vi "Methods to Tree Arr.vi"(7 "Action":T1, 10 "Class":string, 11 "Methods[]":T3(array[cluster])) -> (3 "Properties for Tree Out":T2(array[cluster]))   [LabVIEW 2023] (continued)
Name (localized)"="SceneObject"}, "Method Info"={"Unique ID string"="2d87741e", "Data name"="Light.Set State", "Short name (localized)"="Light.Set State", "Long name (localized)"="Light:Set State"}, "Method Flags"={"IsDeprecated"=FALSE, "IsPrivate"=FALSE, "IsScripting"=FALSE, "IsNotInRun-Time"=FALSE}, "Divider"=FALSE}, {"Class Info"={"Unique ID string"="105", "Parent ID string"="104", "Class Name (unlocalized)"="SceneObject", "Class Name (localized)"="SceneObject"}, "Method Info"={"Unique ID string"="2d87741f", "Data name"="Clip Plane.Get State", "Short name (localized)"="Clip Plane.Get State", "Long name (localized)"="Clip Plane:Get State"}, "Method Flags"={"IsDeprecated"=FALSE, "IsPrivate"=FALSE, "IsScripting"=FALSE, "IsNotInRun-Time"=FALSE}, "Divider"=FALSE}, {"Class Info"={"Unique ID string"="105", "Parent ID string"="104", "Class Name (unlocalized)"="SceneObject", "Class Name (localized)"="SceneObject"}, "Method Info"={"Unique ID string"="2d877420", "Data name"="Clip Plane.Set State", "Short name (localized)"="Clip Plane.Set State", "Long name (localized)"="Clip Plane:Set State"}, "Method Flags"={"IsDeprecated"=FALSE, "IsPrivate"=FALSE, "IsScripting"=FALSE, "IsNotInRun-Time"=FALSE}, "Divider"=FALSE}, {"Class Info"={"Unique ID string"="105", "Parent ID string"="104", "Class Name (unlocalized)"="SceneObject", "Class Name (localized)"="SceneObject"}, "Method Info"={"Unique ID string"="2d877421", "Data name"="Object.Get Object", "Short name (localized)"="Object.Get Object", "Long name (localized)"="Object:Get Object"}, "Method Flags"={"IsDeprecated"=FALSE, "IsPrivate"=FALSE, "IsScripting"=FALSE, "IsNotInRun-Time"=FALSE}, "Divider"=FALSE}, {"Class Info"={"Unique ID string"="105", "Parent ID string"="104", "Class Name (unlocalized)"="SceneObject", "Class Name (localized)"="SceneObject"}, "Method Info"={"Unique ID string"="2d877423", "Data name"="Texture.Set Texture", "Short name (localized)"="Texture.Set Texture", "Long name (localized)"="Texture:Set Texture"}, "Method Flags"={"IsDeprecated"=FALSE, "IsPrivate"=FALSE, "IsScripting"=FALSE, "IsNotInRun-Time"=FALSE}, "Divider"=FALSE}, {"Class Info"={"Unique ID string"="105", "Parent ID string"="104", "Class Name (unlocalized)"="SceneObject", "Class Name (localized)"="SceneObject"}, "Method Info"={"Unique ID string"="2d877424", "Data name"="Texture.RemoveTexture", "Short name (localized)"="Texture.RemoveTexture", "Long name (localized)"="Texture:Remove Texture"}, "Method Flags"={"IsDeprecated"=FALSE, "IsPrivate"=FALSE, "IsScripting"=FALSE, "IsNotInRun-Time"=FALSE}, "Divider"=FALSE}, {"Class Info"={"Unique ID string"="105", "Parent ID string"="104", "Class Name (unlocalized)"="SceneObject", "Class Name (localized)"="SceneObject"}, "Method Info"={"Unique ID string"="2d877425", "Data name"="Light.Add Light", "Short name (localized)"="Light.Add Light", "Long name (localized)"="Light:Add Light"}, "Method Flags"={"IsDeprecated"=FALSE, "IsPrivate"=FALSE, "IsScripting"=FALSE, "IsNotInRun-Time"=FALSE}, "Divider"=FALSE}, {"Class Info"={"Unique ID string"="105", "Parent ID string"="104", "Class Name (unlocalized)"="SceneObject", "Class Name (localized)"="SceneObject"}, "Method Info"={"Unique ID string"="2d877426", "Data name"="Clip Plane.Add Clip Plane", "Short name (localized)"="Clip Plane.Add Clip Plane", "Long name (localized)"="Clip Plane:Add Clip Plane"}, "Method Flags"={"IsDeprecated"=FALSE, "IsPrivate"=FALSE, "IsScripting"=FALSE, "IsNotInRun-Time"=FALSE}, "Divider"=FALSE}, {"Class Info"={"Unique ID string"="105", "Parent ID string"="104", "Class Name (unlocalized)"="SceneObject", "Class Name (localized)"="SceneObject"}, "Method Info"={"Unique ID string"="2d877427", "Data name"="Transformation.Get Rotation", "Short name (localized)"="Transformation.Get Rotation", "Long name (localized)"="Transformation:Get Rotation"}, "Method Flags"={"IsDeprecated"=FALSE, "IsPrivate"=FALSE, "IsScripting"=FALSE, "IsNotInRun-Time"=FALSE}, "Divider"=FALSE}, {"Class Info"={"Unique ID string"="105", "Parent ID string"="104", "Class Name (unlocalized)"="SceneObject", "Class Name (localized)"="SceneObject"}, "Method Info"={"Unique ID string"="2d877428", "Data name"="Transformation.Get Translation", "Short name (localized)"="Transformation.Get Translation", "Long name (localized)"="Transformation:Get Translation"}, "Method Flags"={"IsDeprecated"=FALSE, "IsPrivate"=FALSE, "IsScripting"=FALSE, "IsNotInRun-Time"=FALSE}, "Divider"=FALSE}, {"Class Info"={"Unique ID string"="105", "Parent ID string"="104", "Class Name (unlocalized)"="SceneObject", "Class Name (localized)"="SceneObject"}, "Method Info"={"Unique ID string"="2d877429", "Data name"="Transformation.Get Scale", "Short name (localized)"="Transformation.Get Scale", "Long name (localized)"="Transformation:Get Scale"}, "Method Flags"={"IsDeprecated"=FALSE, "IsPrivate"=FALSE, "IsScripting"=FALSE, "IsNotInRun-Time"=FALSE}, "Divider"=FALSE}, {"Class Info"={"Unique ID string"="105", "Parent ID string"="104", "Class Name (unlocalized)"="SceneObject", "Class Name (localized)"="SceneObject"}, "Method Info"={"Unique ID string"="2d87742a", "Data name"="Light.Get Light", "Short name (localized)"="Light.Get Light", "Long name (localized)"="Light:Get Light"}, "Method Flags"={"IsDeprecated"=FALSE, "IsPrivate"=FALSE, "IsScripting"=FALSE, "IsNotInRun-Time"=FALSE}, "Divider"=FALSE}, {"Class Info"={"Unique ID string"="105", "Parent ID string"="104", "Class Name (unlocalized)"="SceneObject", "Class Name (localized)"="SceneObject"}, "Method Info"={"Unique ID string"="2d87742b", "Data name"="Clip Plane.Get Clip", "Short name (localized)"="Clip Plane.Get Clip", "Long name (localized)"="Clip Plane:Get Clip Plane"}, "Method Flags"={"IsDeprecated"=FALSE, "IsPrivate"=FALSE, "IsScripting"=FALSE, "IsNotInRun-Time"=FALSE}, "Divider"=FALSE}, {"Class Info"={"Unique ID string"="105", "Parent ID string"="104", "Class Name (unlocalized)"="SceneObject", "Class Name (localized)"="SceneObject"}, "Method Info"={"Unique ID string"="2d87742c", "Data name"="Light.Remove Light", "Short name (localized)"="Light.Remove Light", "Long name (localized)"="Light:Remove Light"}, "Method Flags"={"IsDeprecated"=FALSE, "IsPrivate"=FALSE, "IsScripting"=FALSE, "IsNotInRun-Time"=FALSE}, "Divider"=FALSE}, {"Class Info"={"Unique ID string"="105", "Parent ID string"="104", "Class Name (unlocalized)"="SceneObject", "Class Name (localized)"="SceneObject"}, "Method Info"={"Unique ID string"="2d87742d", "Data name"="Clip Plane.Remove Clip", "Short name (localized)"="Clip Plane.Remove Clip", "Long name (localized)"="Clip Plane:Remove Clip Plane"}, "Method Flags"={"IsDeprecated"=FALSE, "IsPrivate"=FALSE, "IsScripting"=FALSE, "IsNotInRun-Time"=FALSE}, "Divider"=FALSE}, {"Class Info"={"Unique ID string"="105", "Parent ID string"="104", "Class Name (unlocalized)"="SceneObject", "Class Name (localized)"="SceneObject"}, "Method Info"={"Unique ID string"="2d87742e", "Data name"="Light.Light Count", "Short name (localized)"="Light.Light Count", "Long name (localized)"="Light:Light Count"}, "Method Flags"={"IsDeprecated"=FALSE, "IsPrivate"=FALSE, "IsScripting"=FALSE, "IsNotInRun-Time"=FALSE}, "Divider"=FALSE}, {"Class Info"={"Unique ID string"="105", "Parent ID string"="104", "Class Name (unlocalized)"="SceneObject", "Class Name (localized)"="SceneObject"}, "Method Info"={"Unique ID string"="2d87742f", "Data name"="Clip Plane.Clip Count", "Short name (localized)"="Clip Plane.Clip Count", "Long name (localized)"="Clip Plane:Clip Plane Count"}, "Method Flags"={"IsDeprecated"=FALSE, "IsPrivate"=FALSE, "IsScripting"=FALSE, "IsNotInRun-Time"=FALSE}, "Divider"=FALSE}, {"Class Info"={"Unique ID string"="105", "Parent ID string"="104", "Class Name (unlocalized)"="SceneObject", "Class Name (localized)"="SceneObject"}, "Method Info"={"Unique ID string"="2d877430", "Data name"="Object.FindObject", "Short name (localized)"="Object.FindObject", "Long name (localized)"="Object:Find Object"}, "Method Flags"={"IsDeprecated"=FALSE, "IsPrivate"=FALSE, "IsScripting"=FALSE, "IsNotInRun-Time"=FALSE}, "Divider"=FALSE}, {"Class Info"={"Unique ID string"="105", "Parent ID string"="104", "Class Name (unlocalized)"="SceneObject", "Class Name (localized)"="SceneObject"}, "Method Info"={"Unique ID string"="2d877431", "Data name"="Set Drawable", "Short name (localized)"="Set Drawable", "Long name (localized)"="Set Drawable"}, "Method Flags"={"IsDeprecated"=FALSE, "IsPrivate"=FALSE, "IsScripting"=FALSE, "IsNotInRun-Time"=FALSE}, "Divider"=FALSE}, {"Class Info"={"Unique ID string"="105", "Parent ID string"="104", "Class Name (unlocalized)"="SceneObject", "Class Name (localized)"="SceneObject"}, "Method Info"={"Unique ID string"="2d877432", "Data name"="SetBillboardParams", "Short name (localized)"="SetBillboardParams", "Long name (localized)"="Set Billboard Params"}, "Method Flags"={"IsDeprecated"=FALSE, "IsPrivate"=FALSE, "IsScripting"=FALSE, "IsNotInRun-Time"=FALSE}, "Divider"=FALSE}, {"Class Info"={"Unique ID string"="105", "Parent ID string"="104", "Class Name (unlocalized)"="SceneObject", "Class Name (localized)"="SceneObject"}, "Method Info"={"Unique ID string"="2d877433", "Data name"="Meshify", "Short name (localized)"="Meshify", "Long name (localized)"="Meshify"}, "Method Flags"={"IsDeprecated"=FALSE, "IsPrivate"=TRUE, "IsScripting"=FALSE, "IsNotInRun-Time"=FALSE}, "Divider"=FALSE}, {"Class Info"={"Unique ID string"="105", "Parent ID string"="104", "Class Name (unlocalized)"="SceneObject", "Class Name (localized)"="SceneObject"}, "Method Info"={"Unique ID string"="2d877434", "Data name"="Bounding.Get Box", "Short name (localized)"="Bounding.Get Box", "Long name (localized)"="Bounding:Get Box"}, "Method Flags"={"IsDeprecated"=FALSE, "IsPrivate"=TRUE, "IsScripting"=FALSE, "IsNotInRun-Time"=FALSE}, "Divider"=FALSE}, {"Class Info"={"Unique ID string"="105", "Parent ID string"="104", "Class Name (unlocalized)"="SceneObject", "Class Name (localized)"="SceneObject"}, "Method Info"={"Unique ID string"="2d877435", "Data name"="Bounding.Get Sphere", "Short name (localized)"="Bounding.Get Sphere", "Long name (localized)"="Bounding:Get Sphere"}, "Method Flags"={"IsDeprecated"=FALSE, "IsPrivate"=TRUE, "IsScripting"=FALSE, "IsNotInRun-Time"=FALSE}, "Divider"=FALSE}, {"Class Info"={"Unique ID string"="111", "Parent ID string"="123", "Class Name (unlocalized)"="SceneTexture", "Class Name (localized)"="SceneTexture"}, "Method Info"={"Unique ID string"="22c3400", "Data name"="Transformation.Rotate", "Short name (localized)"="Transformation.Rotate", "Long name (localized)"="Transformation:Rotate"}, "Method Flags"={"IsDeprecated"=FALSE, "IsPrivate"=FALSE, "IsScripting"=FALSE, "IsNotInRun-Time"=FALSE}, "Divider"=FALSE}, {"Class Info"={"Unique ID string"="111", "Parent ID string"="123", "Class Name (unlocalized)"="SceneTexture", "Class Name (localized)"="SceneTexture"}, "Method Info"={"Unique ID string"="22c3401", "Data name"="Transformation:Translate", "Short name (localized)"="Transformation:Translate", "Long name (localized)"="Transformation:Translate"}, "Method Flags"={"IsDeprecated"=FALSE, "IsPrivate"=FALSE, "IsScripting"=FALSE, "IsNotInRun-Time"=FALSE}, "Divider"=FALSE}, {"Class Info"={"Unique ID string"="111", "Parent ID string"="123", "Class Name (unlocalized)"="SceneTexture", "Class Name (localized)"="SceneTexture"}, "Method Info"={"Unique ID string"="22c3402", "Data name"="Transformation.Scale", "Short name (localized)"="Transformation.Scale", "Long name (localized)"="Transformation:Scale"}, "Method Flags"={"IsDeprecated"=FALSE, "IsPrivate"=FALSE, "IsScripting"=FALSE, "IsNotInRun-Time"=FALSE}, "Divider"=FALSE}, {"Class Info"={"Unique ID string"="111", "Parent ID string"="123", "Class Name (unlocalized)"="SceneTexture", "Class Name (localized)"="SceneTexture"}, "Method Info"={"Unique ID string"="22c3406", "Data name"="Transformation.Clear Transformation", "Short name (localized)"="Transformation.Clear Transformation", "Long name (localized)"="Transformation:Clear Transformation"}, "Method Flags"={"IsDeprecated"=FALSE, "IsPrivate"=FALSE, "IsScripting"=FALSE, "IsNotInRun-Time"=FALSE}, "Divider"=FALSE}, {"Class Info"={"Unique ID string"="111", "Parent ID string"="123", "Class Name (unlocalized)"="SceneTexture", "Class Name (localized)"="SceneTexture"}, "Method Info"={"Unique ID string"="22c3407", "Data name"="Transformation.Set Rotation", "Short name (localized)"="Transformation.Set Rotation", "Long name (localized)"="Transformation:Set Rotation"}, "Method Flags"={"IsDeprecated"=FALSE, "IsPrivate"=FALSE, "IsScripting"=FALSE, "IsNotInRun-Time"=FALSE}, "Divider"=FALSE}, {"Class Info"={"Unique ID string"="111", "Parent ID string"="123", "Class Name (unlocalized)"="SceneTexture", "Class Name (localized)"="SceneTexture"}, "Method Info"={"Unique ID string"="22c3408", "Data name"="Transformation.SetTranslation", "Short name (localized)"="Transformation.SetTranslation", "Long name (localized)"="Transformation:Set Translation"}, "Method Flags"={"IsDeprecated"=FALSE, "IsPrivate"=FALSE, "IsScripting"=FALSE, "IsNotInRun-Time"=FALSE}, "Divider"=FALSE}, {"Class Info"={"Unique ID string"="111", "Parent ID string"="123", "Class Name (unlocalized)"="SceneTexture", "Class Name (localized)"="SceneTexture"}, "Method Info"={"Unique ID string"="22c3409", "Data name"="Transformation.Set Scale", "Short name (localized)"="Transformation.Set Scale", "Long name (localized)"="Transformation:Set Scale"}, "Method Flags"={"IsDeprecated"=FALSE, "IsPrivate"=FALSE, "IsScripting"=FALSE, "IsNotInRun-Time"=FALSE}, "Divider"=FALSE}, {"Class Info"={"Unique ID string"="111", "Parent ID string"="123", "Class Name (unlocalized)"="SceneTexture", "Class Name (localized)"="SceneTexture"}, "Method Info"={"Unique ID string"="22c340a", "Data name"="Transformation.Get Rotation", "Short name (localized)"="Transformation.Get Rotation", "Long name (localized)"="Transformation:Get Rotation"}, "Method Flags"={"IsDeprecated"=FALSE, "IsPrivate"=FALSE, "IsScripting"=FALSE, "IsNotInRun-Time"=FALSE}, "Divider"=FALSE}, {"Class Info"={"Unique ID string"="111", "Parent ID string"="123", "Class Name (unlocalized)"="SceneTexture", "Class Name (localized)"="SceneTexture"}, "Method Info"={"Unique ID string"="22c340b", "Data name"="Transformation.GetTranslation", "Short name (localized)"="Transformation.GetTranslation", "Long name (localized)"="Transformation:Get Translation"}, "Method Flags"={"IsDeprecated"=FALSE, "IsPrivate"=FALSE, "IsScripting"=FALSE, "IsNotInRun-Time"=FALSE}, "Divider"=FALSE}, {"Class Info"={"Unique ID string"="111", "Parent ID string"="123", "Class Name (unlocalized)"="SceneTexture", "Class Name (localized)"="SceneTexture"}, "Method Info"={"Unique ID string"="22c340c", "Data name"="Transformation.Get Scale", "Short name (localized)"="Transformation.Get Scale", "Long name (localized)"="Transformation:Get Scale"}, "Method Flags"={"IsDeprecated"=FALSE, "IsPrivate"=FALSE, "IsScripting"=FALSE, "IsNotInRun-Time"=FALSE}, "Divider"=FALSE}, {"Class Info"={"Unique ID string"="118", "Parent ID string"="112", "Class Name (unlocalized)"="SceneMesh", "Class Name (localized)"="SceneMesh"}, "Method Info"={"Unique ID string"="62a42c00", "Data name"="SetMeshParms", "Short name (localized)"="SetMeshParms", "Long name (localized)"="Set Mesh Parameters"}, "Method Flags"={"IsDeprecated"=FALSE, "IsPrivate"=FALSE, "IsScripting"=FALSE, "IsNotInRun-Time"=FALSE}, "Divider"=FALSE}, {"Class Info"={"Unique ID string"="118", "Parent ID string"="112", "Class Name (unlocalized)"="SceneMesh", "Class Name (localized)"="SceneMesh"}, "Method Info"={"Unique ID string"="62a42c01", "Data name"="ShareArrays", "Short name (localized)"="ShareArrays", "Long name (localized)"="Share Arrays"}, "Method Flags"={"IsDeprecated"=FALSE, "IsPrivate"=FALSE, "IsScripting"=FALSE, "IsNotInRun-Time"=FALSE}, "Divider"=FALSE}, {"Class Info"={"Unique ID string"="118", "Parent ID string"="112", "Class Name (unlocalized)"="SceneMesh", "Class Name (localized)"="SceneMesh"}, "Method Info"={"Unique ID string"="62a42c02", "Data name"="DelaunayMesh", "Short name (localized)"="DelaunayMesh", "Long name (localized)"="Delaunay Mesh"}, "Method Flags"={"IsDeprecated"=FALSE, "IsPrivate"=FALSE, "IsScripting"=FALSE, "IsNotInRun-Time"=FALSE}, "Divider"=FALSE}, {"Class Info"={"Unique ID string"="120", "Parent ID string"="74", "Class Name (unlocalized)"="PropertyFolder", "Class Name (localized)"="PropertyFolder"}, "Method Info"={"Unique ID string"="630d7c00", "Data name"="Add Prop VI", "Short name (localized)"="Add Prop VI", "Long name (localized)"="Add Property VI"}, "Method Flags"={"IsDeprecated"=FALSE, "IsPrivate"=FALSE, "IsScripting"=FALSE, "IsNotInRun-Time"=TRUE}, "Divider"=FALSE}, {"Class Info"={"Unique ID string"="126", "Parent ID string"="80", "Class Name (unlocalized)"="StatechartLibrary", "Class Name (localized)"="StatechartLibrary"}, "Method Info"={"Unique ID string"="18a16402", "Data name"="Generate Code", "Short name (localized)"="Generate Code", "Long name (localized)"="Generate Code"}, "Method Flags"={"IsDeprecated"=FALSE, "IsPrivate"=FALSE, "IsScripting"=FALSE, "IsNotInRun-Time"=TRUE}, "Divider"=FALSE}, {"Class Info"={"Unique ID string"="126", "Parent ID string"="80", "Class Name (unlocalized)"="StatechartLibrary", "Class Name (localized)"="StatechartLibrary"}, "Method Info"={"Unique ID string"="18a16403", "Data name"="Generate Documentation", "Short name (localized)"="Generate Documentation", "Long name (localized)"="Generate Documentation"}, "Method Flags"={"IsDeprecated"=FALSE, "IsPrivate"=FALSE, "IsScripting"=FALSE, "IsNotInRun-Time"=TRUE}, "Divider"=FALSE}, {"Class Info"={"Unique ID string"="129", "Parent ID string"="128", "Class Name (unlocalized)"="SceneText", "Class Name (localized)"="SceneText"}, "Method Info"={"Unique ID string"="c06c00", "Data name"="SetFontName", "Short name (localized)"="SetFontName", "Long name (localized)"="Set Font by Name"}, "Method Flags"={"IsDeprecated"=FALSE, "IsPrivate"=TRUE, "IsScripting"=FALSE, "IsNotInRun-Time"=FALSE}, "Divider"=FALSE}, {"Class Info"={"Unique ID string"="136", "Parent ID string"="6", "Class Name (unlocalized)"="Set", "Class Name (localized)"="Set"}, "Method Info"={"Unique ID string"="4e878c00", "Data name"="ScrollToElement", "Short name (localized)"="ScrollToElement", "Long name (localized)"="Scroll to Element"}, "Method Flags"={"IsDeprecated"=FALSE, "IsPrivate"=FALSE, "IsScripting"=FALSE, "IsNotInRun-Time"=FALSE}, "Divider"=FALSE}, {"Class Info"={"Unique ID string"="137", "Parent ID string"="6", "Class Name (unlocalized)"="Map", "Class Name (localized)"="Map"}, "Method Info"={"Unique ID string"="16099400", "Data name"="ScrollToKey", "Short name (localized)"="ScrollToKey", "Long name (localized)"="Scroll To Key"}, "Method Flags"={"IsDeprecated"=FALSE, "IsPrivate"=FALSE, "IsScripting"=FALSE, "IsNotInRun-Time"=FALSE}, "Divider"=FALSE}, {"Class Info"={"Unique ID string"="16384", "Parent ID string"="16503", "Class Name (unlocalized)"="Diagram", "Class Name (localized)"="Diagram"}, "Method Info"={"Unique ID string"="6d17c800", "Data name"="ObjectFromPoint", "Short name (localized)"="ObjectFromPoint", "Long name (localized)"="Object From Point"}, "Method Flags"={"IsDeprecated"=FALSE, "IsPrivate"=TRUE, "IsScripting"=TRUE, "IsNotInRun-Time"=FALSE}, "Divider"=FALSE}, {"Class Info"={"Unique ID string"="16384", "Parent ID string"="16503", "Class Name (unlocalized)"="Diagram", "Class Name (localized)"="Diagram"}, "Method Info"={"Unique ID string"="6d17c801", "Data name"="CleanUp", "Short name (localized)"="CleanUp", "Long name (localized)"="Clean Up Diagram"}, "Method Flags"={"IsDeprecated"=FALSE, "IsPrivate"=FALSE, "IsScripting"=TRUE, "IsNotInRun-Time"=FALSE}, "Divider"=FALSE}, {"Class Info"={"Unique ID string"="16384", "Parent ID string"="16503", "Class Name (unlocalized)"="Diagram", "Class Name (localized)"="Diagram"}, "Method Info"={"Unique ID string"="6d17c802", "Data name"="CleanUpOptions", "Short name (localized)"="CleanUpOptions", "Long name (localized)"="Default Diagram Clean Up Options"}, "Method Flags"={"IsDeprecated"=FALSE, "IsPrivate"=FALSE, "IsScripting"=TRUE, "IsNotInRun-Time"=FALSE}, "Divider"=FALSE}, {"Class Info"={"Unique ID string"="16384", "Parent ID string"="16503", "Class Name (unlocalized)"="Diagram", "Class Name (localized)"="Diagram"}, "Method Info"={"Unique ID string"="6d17c804", "Data name"="Create from Data Type", "Short name (localized)"="Create from Data Type", "Long name (localized)"="Create from Data Type"}, "Method Flags"={"IsDeprecated"=FALSE, "IsPrivate"=FALSE, "IsScripting"=TRUE, "IsNotInRun-Time"=TRUE}, "Divider"=FALSE}, {"Class Info"={"Unique ID string"="16385", "Parent ID string"="36", "Class Name (unlocalized)"="Terminal", "Class Name (localized)"="Terminal"}, "Method Info"={"Unique ID string"="6349c00", "Data name"="Create Constant", "Short name (localized)"="Create Constant", "Long name (localized)"="Create Constant"}, "Method Flags"={"IsDeprecated"=FALSE, "IsPrivate"=FALSE, "IsScripting"=TRUE, "IsNotInRun-Time"=TRUE}, "Divider"=FALSE}, {"Class Info"={"Unique ID string"="16385", "Parent ID string"="36", "Class Name (unlocalized)"="Terminal", "Class Name (localized)"="Terminal"}, "Method Info"={"Unique ID string"="6349c01", "Data name"="Create Control", "Short name (localized)"="Create Control", "Long name (localized)"="Create Control"}, "Method Flags"={"IsDeprecated"=FALSE, "IsPrivate"=FALSE, "IsScripting"=TRUE, "IsNotInRun-Time"=TRUE}, "Divider"=FALSE}, {"Class Info"={"Unique ID string"="16385", "Parent ID string"="36", "Class Name (unlocalized)"="Terminal", "Class Name (localized)"="Terminal"}, "Method Info"={"Unique ID string"="6349c02", "Data name"="Create Indicator", "Short name (localized)"="Create Indicator", "Long name (localized)"="Create Indicator"}, "Method Flags"={"IsDeprecated"=FALSE, "IsPrivate"=FALSE, "IsScripting"=TRUE, "IsNotInRun-Time"=TRUE}, "Divider"=FALSE}, {"Class Info"={"Unique ID string"="16385", "Parent ID string"="36", "Class Name (unlocalized)"="Terminal", "Class Name (localized)"="Terminal"}, "Method Info"={"Unique ID string"="6349c03", "Data name"="Connect Wire", "Short name (localized)"="Connect Wire", "Long name (localized)"="Connect Wire"}, "Method Flags"={"IsDeprecated"=FALSE, "IsPrivate"=FALSE, "IsScripting"=TRUE, "IsNotInRun-Time"=TRUE}, "Divider"=FALSE}, {"Class Info"={"Unique ID string"="16385", "Parent ID string"="36", "Class Name (unlocalized)"="Terminal", "Class Name (localized)"="Terminal"}, "Method Info"={"Unique ID string"="6349c04", "Data name"="Create Described Wire", "Short name (localized)"="Create Described Wire", "Long name (localized)"="Create Described Wire"}, "Method Flags"={"IsDeprecated"=FALSE, "IsPrivate"=FALSE, "IsScripting"=TRUE, "IsNotInRun-Time"=TRUE}, "Divider"=FALSE}, {"Class Info"={"Unique ID string"="16385", "Parent ID string"="36", "Class Name (unlocalized)"="Terminal", "Class Name (localized)"="Terminal"}, "Method Info"={"Unique ID string"="6349c05", "Data name"="Create Shared Variable Node", "Short name (localized)"="Create Shared Variable Node", "Long name (localized)"="Create Shared Variable Node"}, "Method Flags"={"IsDeprecated"=FALSE, "IsPrivate"=FALSE, "IsScripting"=TRUE, "IsNotInRun-Time"=TRUE}, "Divider"=FALSE}, {"Class Info"={"Unique ID string"="16386", "Parent ID string"="36", "Class Name (unlocalized)"="Constant", "Class Name (localized)"="Constant"}, "Method Info"={"Unique ID string"="634a800", "Data name"="Discon Typedef", "Short name (localized)"="Discon Typedef", "Long name (localized)"="Disconnect From Typedef"}, "Method Flags"={"IsDeprecated"=FALSE, "IsPrivate"=FALSE, "IsScripting"=TRUE, "IsNotInRun-Time"=TRUE}, "Divider"=FALSE}, {"Class Info"={"Unique ID string"="16386", "Parent ID string"="36", "Class Name (unlocalized)"="Constant", "Class Name (localized)"="Constant"}, "Method Info"={"Unique ID string"="634a801", "Data name"="Update Typedef", "Short name (localized)"="Update Typedef", "Long name (localized)"="Update From Typedef"}, "Method Flags"={"IsDeprecated"=FALSE, "IsPrivate"=FALSE, "IsScripting"=TRUE, "IsNotInRun-Time"=TRUE}, "Divider"=FALSE}, {"Class Info"={"Unique ID string"="16386", "Parent ID string"="36", "Class Name (unlocalized)"="Constant", "Class Name (localized)"="Constant"}, "Method Info"={"Unique ID string"="634a802", "Data name"="Change to Control", "Short name (localized)"="Change to Control", "Long name (localized)"="Change to Control"}, "Method Flags"={"IsDeprecated"=FALSE, "IsPrivate"=FALSE, "IsScripting"=TRUE, "IsNotInRun-Time"=TRUE}, "Divider"=FALSE}, {"Class Info"={"Unique ID string"="16386", "Parent ID string"="36", "Class Name (unlocalized)"="Constant", "Class Name (localized)"="Constant"}, "Method Info"={"Unique ID string"="634a803", "Data name"="Change to Indicator", "Short name (localized)"="Change to Indicator", "Long name (localized)"="Change to Indicator"}, "Method Flags"={"IsDeprecated"=FALSE, "IsPrivate"=FALSE, "IsScripting"=TRUE, "IsNotInRun-Time"=TRUE}, "Divider"=FALSE}, {"Class Info"={"Unique ID string"="16386", "Parent ID string"="36", "Class Name (unlocalized)"="Constant", "Class Name (localized)"="Constant"}, "Method Info"={"Unique ID string"="634a804", "Data name"="Copy Data", "Short name (localized)"="Copy Data", "Long name (localized)"="Copy Data"}, "Method Flags"={"IsDeprecated"=FALSE, "IsPrivate"=FALSE, "IsScripting"=TRUE, "IsNotInRun-Time"=TRUE}, "Divider"=FALSE}, {"Class Info"={"Unique ID string"="16386", "Parent ID string"="36", "Class Name (unlocalized)"="Constant", "Class Name (localized)"="Constant"}, "Method Info"={"Unique ID string"="634a806", "Data name"="Paste Data", "Short name (localized)"="Paste Data", "Long name (localized)"="Paste Data"}, "Method Flags"={"IsDeprecated"=FALSE, "IsPrivate"=FALSE, "IsScripting"=TRUE, "IsNotInRun-Time"=TRUE}, "Divider"=FALSE}, {"Class Info"={"Unique ID string"="16386", "Parent ID string"="36", "Class Name (unlocalized)"="Constant", "Class Name (localized)"="Constant"}, "Method Info"={"Unique ID string"="634a807", "Data name"="Change to Shared Variable Node", "Short name (localized)"="Change to Shared Variable Node", "Long name (localized)"="Change to Shared Variable Node"}, "Method Flags"={"IsDeprecated"=FALSE, "IsPrivate"=FALSE, "IsScripting"=TRUE, "IsNotInRun-Time"=TRUE}, "Divider"=FALSE}, {"Class Info"={"Unique ID string"="16388", "Parent ID string"="16386", "Class Name (unlocalized)"="ArrayConstant", "Class Name (localized)"="ArrayConstant"}, "Method Info"={"Unique ID string"="634c000", "Data name"="Empty Array", "Short name (localized)"="Empty Array", "Long name (localized)"="Empty Array"}, "Method Flags"={"IsDeprecated"=FALSE, "IsPrivate"=FALSE, "IsScripting"=TRUE, "IsNotInRun-Time"=FALSE}, "Divider"=FALSE}, {"Class Info"={"Unique ID string"="16388", "Parent ID string"="16386", "Class Name (unlocalized)"="ArrayConstant", "Class Name (localized)"="ArrayConstant"}, "Method Info"={"Unique ID string"="634c001", "Data name"="Insert Row Before", "Short name (localized)"="Insert Row Before", "Long name (localized)"="Insert Row Before"}, "Method Flags"={"IsDeprecated"=FALSE, "IsPrivate"=FALSE, "IsScripting"=TRUE, "IsNotInRun-Time"=FALSE}, "Divider"=FALSE}, {"Class Info"={"Unique ID string"="16388", "Parent ID string"="16386", "Class Name (unlocalized)"="ArrayConstant", "Class Name (localized)"="ArrayConstant"}, "Method Info"={"Unique ID string"="634c002", "Data name"="Insert Column Before", "Short name (localized)"="Insert Column Before", "Long name (localized)"="Insert Column Before"}, "Method Flags"={"IsDeprecated"=FALSE, "IsPrivate"=FALSE, "IsScripting"=TRUE, "IsNotInRun-Time"=FALSE}, "Divider"=FALSE}, {"Class Info"={"Unique ID string"="16388", "Parent ID string"="16386", "Class Name (unlocalized)"="ArrayConstant", "Class Name (localized)"="ArrayConstant"}, "Method Info"={"Unique ID string"="634c003", "Data name"="Delete Row", "Short name (localized)"="Delete Row", "Long name (localized)"="Delete Row"}, "Method Flags"={"IsDeprecated"=FALSE, "IsPrivate"=FALSE, "IsScripting"=TRUE, "IsNotInRun-Time"=FALSE}, "Divider"=FALSE}, {"Class Info"={"Unique ID string"="16388", "Parent ID string"="16386", "Class Name (unlocalized)"="ArrayConstant", "Class Name (localized)"="ArrayConstant"}, "Method Info"={"Unique ID string"="634c004", "Data name"="Delete Column", "Short name (localized)"="Delete Column", "Long name (localized)"="Delete Column"}, "Method Flags"={"IsDeprecated"=FALSE, "IsPrivate"=FALSE, "IsScripting"=TRUE, "IsNotInRun-Time"=FALSE}, "Divider"=FALSE}, {"Class Info"={"Unique ID string"="16388", "Parent ID string"="16386", "Class Name (unlocalized)"="ArrayConstant", "Class Name (localized)"="ArrayConstant"}, "Method Info"={"Unique ID string"="634c005", "Data name"="Insert Element Before", "Short name (localized)"="Insert Element Before", "Long name (localized)"="Insert Element Before"}, "Method Flags"={"IsDeprecated"=FALSE, "IsPrivate"=FALSE, "IsScripting"=TRUE, "IsNotInRun-Time"=FALSE}, "Divider"=FALSE}, {"Class Info"={"Unique ID string"="16388", "Parent ID string"="16386", "Class Name (unlocalized)"="ArrayConstant", "Class Name (localized)"="ArrayConstant"}, "Method Info"={"Unique ID string"="634c006", "Data name"="Delete Element", "Short name (localized)"="Delete Element", "Long name (localized)"="Delete Element"}, "Method Flags"={"IsDeprecated"=FALSE, "IsPrivate"=FALSE, "IsScripting"=TRUE, "IsNotInRun-Time"=FALSE}, "Divider"=FALSE}, {"Class Info"={"Unique ID string"="16393", "Parent ID string"="16386", "Class Name (unlocalized)"="ClusterConstant", "Class Name (localized)"="ClusterConstant"}, "Method Info"={"Unique ID string"="6350800", "Data name"="Auto Size", "Short name (localized)"="Auto Size", "Long name (localized)"="Auto Size"}, "Method Flags"={"IsDeprecated"=FALSE, "IsPrivate"=FALSE, "IsScripting"=TRUE, "IsNotInRun-Time"=TRUE}, "Divider"=FALSE}, {"Class Info"={"Unique ID string"="16393", "Parent ID string"="16386", "Class Name (unlocalized)"="ClusterConstant", "Class Name (localized)"="ClusterConstant"}, "Method Info"={"Unique ID string"="6350801", "Data name"="ReorderElements", "Short name (localized)"="ReorderElements", "Long name (localized)"="ReorderElements"}, "Method Flags"={"IsDeprecated"=FALSE, "IsPrivate"=FALSE, "IsScripting"=TRUE, "IsNotInRun-Time"=FALSE}, "Divider"=FALSE}, {"Class Info"={"Unique ID string"="16395", "Parent ID string"="16385", "Class Name (unlocalized)"="ControlTerminal", "Class Name (localized)"="ControlTerminal"}, "Method Info"={"Unique ID string"="6352c00", "Data name"="Toggle Direction", "Short name (localized)"="Toggle Direction", "Long name (localized)"="Toggle Direction"}, "Method Flags"={"IsDeprecated"=FALSE, "IsPrivate"=FALSE, "IsScripting"=TRUE, "IsNotInRun-Time"=FALSE}, "Divider"=FALSE}, {"Class Info"={"Unique ID string"="16395", "Parent ID string"="16385", "Class Name (unlocalized)"="ControlTerminal", "Class Name (localized)"="ControlTerminal"}, "Method Info"={"Unique ID string"="6352c01", "Data name"="Change To Constant", "Short name (localized)"="Change To Constant", "Long name (localized)"="Change To Constant"}, "Method Flags"={"IsDeprecated"=FALSE, "IsPrivate"=FALSE, "IsScripting"=TRUE, "IsNotInRun-Time"=FALSE}, "Divider"=FALSE}, {"Class Info"={"Unique ID string"="16395", "Parent ID string"="16385", "Class Name (unlocalized)"="ControlTerminal", "Class Name (localized)"="ControlTerminal"}, "Method Info"={"Unique ID string"="6352c02", "Data name"="Change to Shared Variable Node", "Short name (localized)"="Change to Shared Variable Node", "Long name (localized)"="Change to Shared Variable Node"}, "Method Flags"={"IsDeprecated"=FALSE, "IsPrivate"=FALSE, "IsScripting"=TRUE, "IsNotInRun-Time"=TRUE}, "Divider"=FALSE}, {"Class Info"={"Unique ID string"="16397", "Parent ID string"="16421", "Class Name (unlocalized)"="Global", "Class Name (localized)"="Global"}, "Method Info"={"Unique ID string"="6354400", "Data name"="Relink To VI", "Short name (localized)"="Relink To VI", "Long name (localized)"="Relink To VI"}, "Method Flags"={"IsDeprecated"=FALSE, "IsPrivate"=FALSE, "IsScripting"=TRUE, "IsNotInRun-Time"=TRUE}, "Divider"=FALSE}, {"Class Info"={"Unique ID string"="16401", "Parent ID string"="16421", "Class Name (unlocalized)"="SubVI", "Class Name (localized)"="SubVI"}, "Method Info"={"Unique ID string"="635e000", "Data name"="Relink To VI", "Short name (localized)"="Relink To VI", "Long name (localized)"="Relink To VI"}, "Method Flags"={"IsDeprecated"=FALSE, "IsPrivate"=FALSE, "IsScripting"=TRUE, "IsNotInRun-Time"=TRUE}, "Divider"=FALSE}, {"Class Info"={"Unique ID string"="16401", "Parent ID string"="16421", "Class Name (unlocalized)"="SubVI", "Class Name (localized)"="SubVI"}, "Method Info"={"Unique ID string"="635e001", "Data name"="Replace", "Short name (localized)"="Replace", "Long name (localized)"="Replace"}, "Method Flags"={"IsDeprecated"=FALSE, "IsPrivate"=TRUE, "IsScripting"=TRUE, "IsNotInRun-Time"=TRUE}, "Divider"=FALSE}, {"Class Info"={"Unique ID string"="16401", "Parent ID string"="16421", "Class Name (unlocalized)"="SubVI", "Class Name (localized)"="SubVI"}, "Method Info"={"Unique ID string"="635e002", "Data name"="Inline", "Short name (localized)"="Inline", "Long name (localized)"="Inline"}, "Method Flags"={"IsDeprecated"=FALSE, "IsPrivate"=FALSE, "IsScripting"=TRUE, "IsNotInRun-Time"=FALSE}, "Divider"=FALSE}, {"Class Info"={"Unique ID string"="16401", "Parent ID string"="16421", "Class Name (unlocalized)"="SubVI", "Class Name (localized)"="SubVI"}, "Method Info"={"Unique ID string"="635e003", "Data name"="Feeds Through", "Short name (localized)"="Feeds Through", "Long name (localized)"="Feeds Through"}, "Method Flags"={"IsDeprecated"=FALSE, "IsPrivate"=TRUE, "IsScripting"=TRUE, "IsNotInRun-Time"=FALSE}, "Divider"=FALSE}, {"Class Info"={"Unique ID string"="16401", "Parent ID string"="16421", "Class Name (unlocalized)"="SubVI", "Class Name (localized)"="SubVI"}, "Method Info"={"Unique ID string"="635e004", "Data name"="SwapInstanceVI", "Short name (localized)"="SwapInstanceVI", "Long name (localized)"="Swap Instance VI"}, "Method Flags"={"IsDeprecated"=FALSE, "IsPrivate"=TRUE, "IsScripting"=TRUE, "IsNotInRun-Time"=TRUE}, "Divider"=FALSE}, {"Class Info"={"Unique ID string"="16402", "Parent ID string"="16421", "Class Name (unlocalized)"="CallByRef", "Class Name (localized)"="CallByRef"}, "Method Info"={"Unique ID string"="635ec00", "Data name"="Configure", "Short name (localized)"="Configure", "Long name (localized)"="Configure"}, "Method Flags"={"IsDeprecated"=FALSE, "IsPrivate"=TRUE, "IsScripting"=TRUE, "IsNotInRun-Time"=FALSE}, "Divider"=FALSE}, {"Class Info"={"Unique ID string"="16402", "Parent ID string"="16421", "Class Name (unlocalized)"="CallByRef", "Class Name (localized)"="CallByRef"}, "Method Info"={"Unique ID string"="635ec01", "Data name"="ConvertStartAsyncCall", "Short name (localized)"="ConvertStartAsyncCall", "Long name (localized)"="Convert:Start Asynchronous Call"}, "Method Flags"={"IsDeprecated"=FALSE, "IsPrivate"=FALSE, "IsScripting"=TRUE, "IsNotInRun-Time"=TRUE}, "Divider"=FALSE}, {"Class Info"={"Unique ID string"="16402", "Parent ID string"="16421", "Class Name (unlocalized)"="CallByRef", "Class Name (localized)"="CallByRef"}, "Method Info"={"Unique ID string"="635ec02", "Data name"="ConvertWaitAsyncCall", "Short name (localized)"="ConvertWaitAsyncCall", "Long name (localized)"="Convert:Wait On Asynchronous Call"}, "Method Flags"={"IsDeprecated"=FALSE, "IsPrivate"=FALSE, "IsScripting"=TRUE, "IsNotInRun-Time"=TRUE}, "Divider"=FALSE}, {"Class Info"={"Unique ID string"="16402", "Parent ID string"="16421", "Class Name (unlocalized)"="CallByRef", "Class Name (localized)"="CallByRef"}, "Method Info"={"Unique ID string"="635ec03", "Data name"="ConvertCallByRef", "Short name (localized)"="ConvertCallByRef", "Long name (localized)"="Convert:Call By Reference"}, "Method Flags"={"IsDeprecated"=FALSE, "IsPrivate"=FALSE, "IsScripting"=TRUE, "IsNotInRun-Time"=TRUE}, "Divider"=FALSE}, {"Class Info"={"Unique ID string"="16404", "Parent ID string"="16421", "Class Name (unlocalized)"="Structure", "Class Name (localized)"="Structure"}, "Method Info"={"Unique ID string"="6360400", "Data name"="Auto Size", "Short name (localized)"="Auto Size", "Long name (localized)"="Auto Size"}, "Method Flags"={"IsDeprecated"=FALSE, "IsPrivate"=FALSE, "IsScripting"=TRUE, "IsNotInRun-Time"=TRUE}, "Divider"=FALSE}, {"Class Info"={"Unique ID string"="16404", "Parent ID string"="16421", "Class Name (unlocalized)"="Structure", "Class Name (localized)"="Structure"}, "Method Info"={"Unique ID string"="6360401", "Data name"="Remove Structure", "Short name (localized)"="Remove Structure", "Long name (localized)"="Remove Structure"}, "Method Flags"={"IsDeprecated"=FALSE, "IsPrivate"=FALSE, "IsScripting"=TRUE, "IsNotInRun-Time"=TRUE}, "Divider"=FALSE}, {"Class Info"={"Unique ID string"="16404", "Parent ID string"="16421", "Class Name (unlocalized)"="Structure", "Class Name (localized)"="Structure"}, "Method Info"={"Unique ID string"="6360402", "Data name"="PreAllocSharedClones", "Short name (localized)"="PreAllocSharedClones", "Long name (localized)"="Shared Clones:Pre-Allocate"}, "Method Flags"={"IsDeprecated"=FALSE, "IsPrivate"=FALSE, "IsScripting"=TRUE, "IsNotInRun-Time"=FALSE}, "Divider"=FALSE}, {"Class Info"={"Unique ID string"="16404", "Parent ID string"="16421", "Class Name (unlocalized)"="Structure", "Class Name (localized)"="Structure"}, "Method Info"={"Unique ID string"="6360403", "Data name"="AllocSharedClonesAsNeeded", "Short name (localized)"="AllocSharedClonesAsNeeded", "Long name (localized)"="Shared Clones:Allocate as Needed"}, "Method Flags"={"IsDeprecated"=FALSE, "IsPrivate"=FALSE, "IsScripting"=TRUE, "IsNotInRun-Time"=FALSE}, "Divider"=FALSE}, {"Class Info"={"Unique ID string"="16405", "Parent ID string"="16404", "Class Name (unlocalized)"="Loop", "Class Name (localized)"="Loop"}, "Method Info"={"Unique ID string"="6361000", "Data name"="Add Shift Register", "Short name (localized)"="Add Shift Register", "Long name (localized)"="Add Shift Register"}, "Method Flags"={"IsDeprecated"=FALSE, "IsPrivate"=FALSE, "IsScripting"=TRUE, "IsNotInRun-Time"=TRUE}, "Divider"=FALSE}, {"Class Info"={"Unique ID string"="16406", "Parent ID string"="16404", "Class Name (unlocalized)"="MultiFrameStructure", "Class Name (localized)"="MultiFrameStructure"}, "Method Info"={"Unique ID string"="6363400", "Data name"="Add Frame", "Short name (localized)"="Add Frame", "Long name (localized)"="Add Frame"}, "Method Flags"={"IsDeprecated"=FALSE, "IsPrivate"=FALSE, "IsScripting"=TRUE, "IsNotInRun-Time"=TRUE}, "Divider"=FALSE}, {"Class Info"={"Unique ID string"="16406", "Parent ID string"="16404", "Class Name (unlocalized)"="MultiFrameStructure", "Class Name (localized)"="MultiFrameStructure"}, "Method Info"={"Unique ID string"="6363401", "Data name"="Remove Frame", "Short name (localized)"="Remove Frame", "Long name (localized)"="Remove Frame"}, "Method Flags"={"IsDeprecated"=FALSE, "IsPrivate"=FALSE, "IsScripting"=TRUE, "IsNotInRun-Time"=TRUE}, "Divider"=FALSE}, {"Class Info"={"Unique ID string"="16406", "Parent ID string"="16404", "Class Name (unlocalized)"="MultiFrameStructure", "Class Name (localized)"="MultiFrameStructure"}, "Method Info"={"Unique ID string"="6363402", "Data name"="Duplicate Frame", "Short name (localized)"="Duplicate Frame", "Long name (localized)"="Duplicate Frame"}, "Method Flags"={"IsDeprecated"=FALSE, "IsPrivate"=FALSE, "IsScripting"=TRUE, "IsNotInRun-Time"=TRUE}, "Divider"=FALSE}, {"Class Info"={"Unique ID string"="16406", "Parent ID string"="16404", "Class Name (unlocalized)"="MultiFrameStructure", "Class Name (localized)"="MultiFrameStructure"}, "Method Info"={"Unique ID string"="6363403", "Data name"="RearrangeFramesByIdx", "Short name (localized)"="RearrangeFramesByIdx", "Long name (localized)"="Rearrange Frames By Index"}, "Method Flags"={"IsDeprecated"=FALSE, "IsPrivate"=FALSE, "IsScripting"=TRUE, "IsNotInRun-Time"=FALSE}, "Divider"=FALSE}, {"Class Info"={"Unique ID string"="16406", "Parent ID string"="16404", "Class Name (unlocalized)"="MultiFrameStructure", 
